vi "U16_to_FrameName.vi"(3 "u16":u16) -> (1 "FrameName":string)   [LabVIEW 2019, in "BlueSerializationScripts.lvlib"]
uses:
  BlueSerializationScripts.lvlib
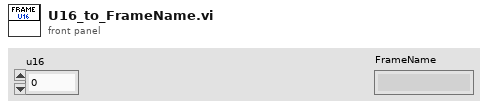
[diagram p1: front panel]
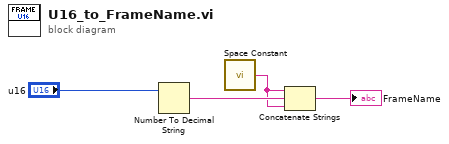
[diagram p0: block diagram]
diagram:
  n1 = Number To Decimal String(number="u16") -> (decimal integer string=w3:string)  [unwired: 1 in]
  n2 = call <vilib>:"Space Constant.vi"() -> ("String"=w2:string)
  n3 = Concatenate Strings(w2, w3, w2) -> (→"FrameName":string)
